vi "Test Permutate 4 chars.vi"(11 "Test Case In":refnum<class "Path Permutation Test.lvclass">) -> (0 "error out":errorcluster, 3 "Test Case Out":refnum<class "Path Permutation Test.lvclass">)   [LabVIEW 2020, in "Path Permutation Test.lvclass"]
uses:
  Path Permutation Test.lvclass
  C:/Program Files (x86)/National Instruments/LabVIEW 2020/vi.lib/Astemes/LUnit/Test Case.lvclass
  <vilib>/Astemes/LUnit/Test Case.lvclass/Test Case.ctl
  4b4b7a30-a351-49c7-bde2-d192d5c541ae.vi
  <vilib>/Astemes/LUnit/Palette/Pass If.vi
  <vilib>/Astemes/LUnit/Append Fail Result.vi
  <vilib>/Astemes/LUnit/Append Pass Result.vi
  <vilib>/Astemes/LUnit/Run In UI.vi
  <vilib>/Utility/error.llb/Clear Errors.vi
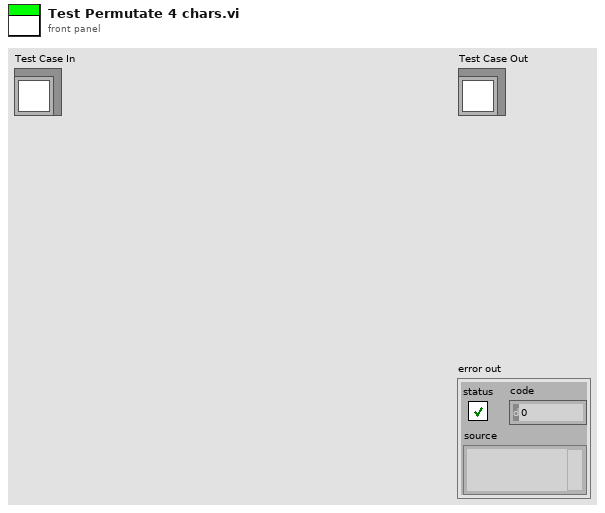
[diagram p1: front panel]
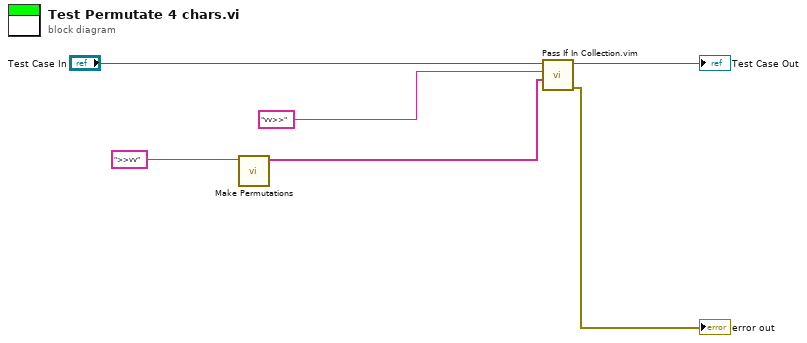
[diagram p0: block diagram]
diagram:
  n1 = call "Make Permutations.vi"("String"=">>vv") -> ("Array"=w3:string[])  [unwired: 10 in]
  n2 = call "Pass If In Collection.vim"("Collection"=w3, "Expected Element"="vv>>", "LUnit Test Case In"="Test Case In") -> ("error out"=→"error out":errorcluster, "LUnit Test Case Out"=→"Test Case Out":refnum<class "Path Permutation Test.lvclass">)  [unwired: 7 in]
